vi "Engine-Event-WindowMoved.vi"(6 "Y":i32, 8 "error in (no error)":errorcluster, 9 "X":i32, 10 "Timestamp":u64, 11 "GLF Window in":refnum<class "Window.lvclass">) -> (0 "error out":errorcluster, 3 "GLF Window out":refnum<class "Window.lvclass">)   [LabVIEW 2020, in "GLF.lvlib" / "Window.lvclass"]
uses:
  Window.lvclass
  Window.lvclass/Window.ctl
  WindowEventInterface/WindowEventInterface.lvclass
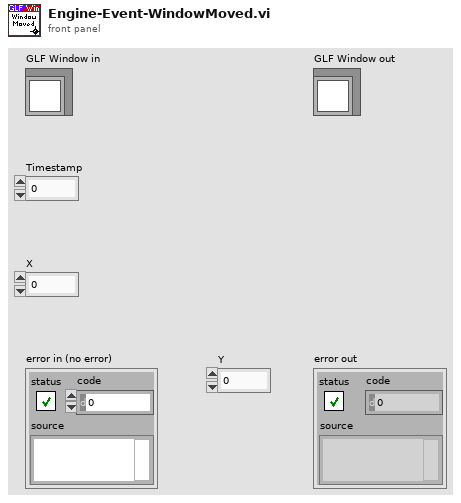
[diagram p1: front panel]
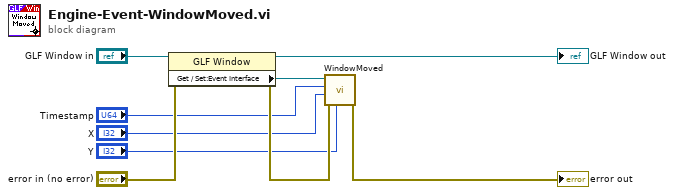
[diagram p0: block diagram]
diagram:
  n1 = property class="GLF Window"(reference="GLF Window in", error in="error in (no error)") -> (reference out=→"GLF Window out":refnum<class "Window.lvclass">, error out=w5:errorcluster, "Get / Set:Event Interface"=w6:refnum<class "WindowEventInterface.lvclass">)
  n2 = call-dynamic "WindowMoved.vi"("Y"="Y", "error in (no error)"=w5, "X"="X", "Timestamp"="Timestamp", "WindowEventInterface in"=w6) -> ("error out"=→"error out":errorcluster)  [unwired: 6 in]
